vi "Read_INI.vi"(3 "error in (no error)":errorcluster caption="错误输入（无错误）") -> (0 "error out":errorcluster caption="错误输出", 2 "HandsPara":T1)   [LabVIEW 2016]
uses:
  Controls/handspara.ctl
  <vilib>/Utility/config.llb/Read Key (U32).vi
  <vilib>/Utility/config.llb/NI_LVConfig.lvlib
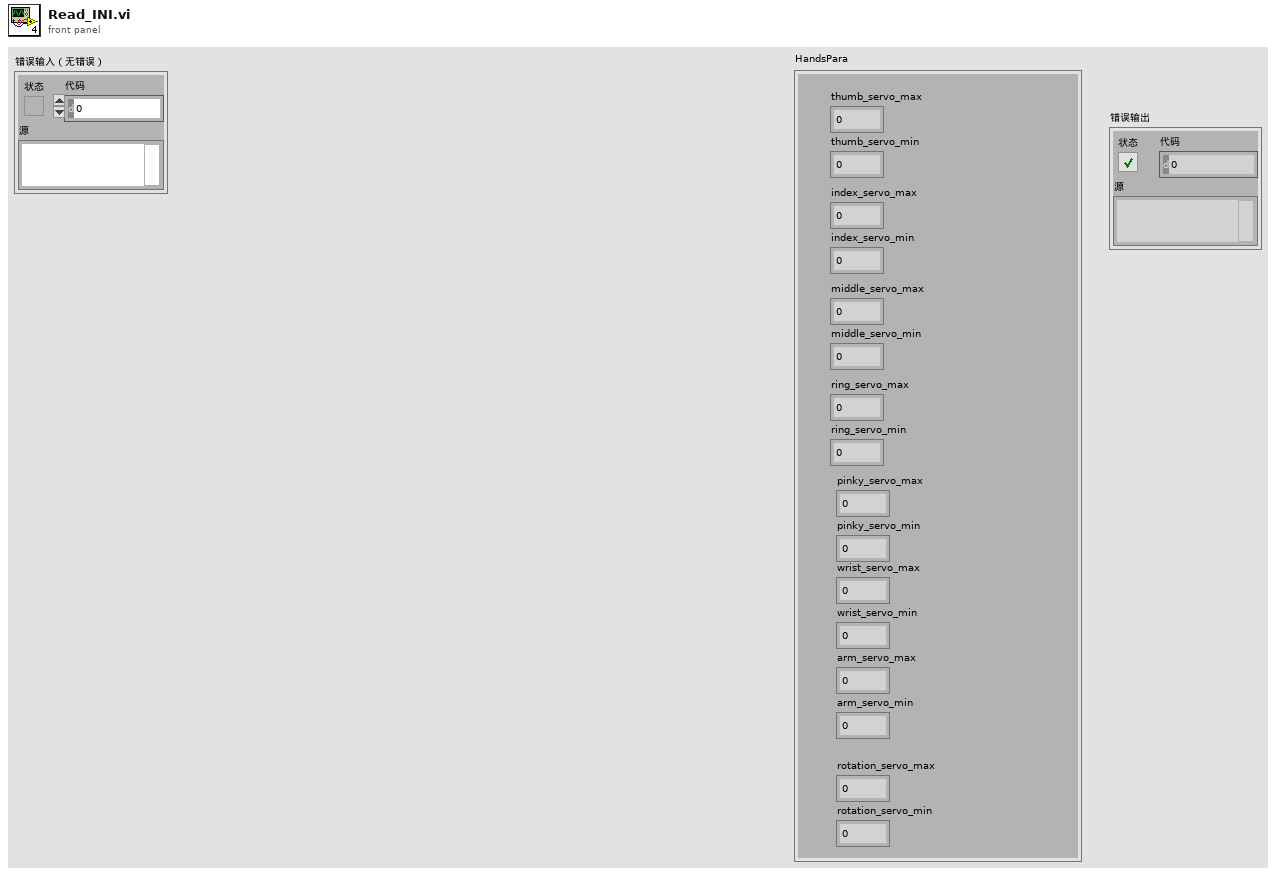
[diagram p1: front panel]
types:
  T1 = typedef "handspara.ctl" = cluster{"thumb_servo_max":u32, "thumb_servo_min":u32, "index_servo_max ":u32, "index_servo_min":u32, "middle_servo_max ":u32, "middle_servo_min":u32, "ring_servo_max":u32, "ring_servo_min":u32, "pinky_servo_max ":u32, "pinky_servo_min ":u32, "wrist_servo_max":u32, "wrist_servo_min":u32, "arm_servo_max ":u32, "arm_servo_min":u32, "rotation_servo_max ":u32, "rotation_servo_min ":u32}
  T2 = typedef "NI_LVConfig.lvlib/Config Data RefNum.ctl" = refnum<k1>
  T3 = cluster{"[0]":u32, "[1]":u32, "[2]":u32, "[3]":u32, "[4]":u32, "[5]":u32, "[6]":u32, "[7]":u32, "[8]":u32, "[9]":u32, "[10]":u32, "[11]":u32, "[12]":u32, "[13]":u32, "[14]":u32, "[15]":u32}
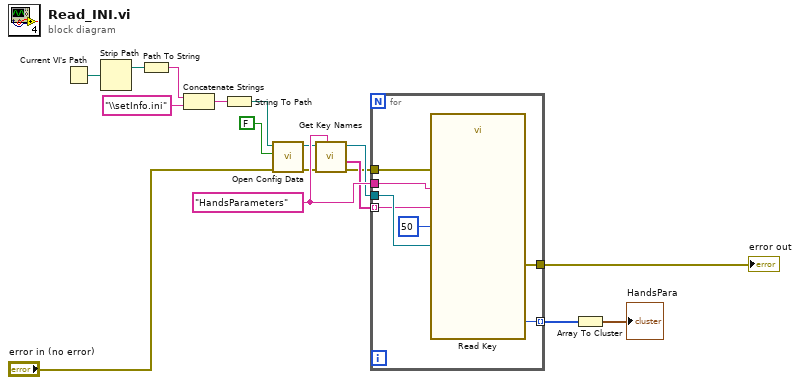
[diagram p0: block diagram]
diagram:
  w10 = "HandsParameters" ("section")
  n1 = Current VI's Path() -> (path=w15:path)
  n2 = Strip Path(path=w15) -> (stripped path=w14:path)  [unwired: 1 out]
  n3 = Path To String(path=w14) -> (string=w17:string)
  n4 = Concatenate Strings(w17, "\\setInfo.ini" ("string")) -> (w16:string)
  n5 = String To Path(string=w16) -> (path=w11:path)
  n6 = call <vilib>:"Open Config Data.vi"("error in (no error)"="error in (no error)", "create file if necessary (T)"=FALSE, "configuration file path"=w11) -> ("error out"=w6:errorcluster, "refnum"=w8:T2)  [unwired: 6 in, 1 out]
  n7 = call <vilib>:"Get Key Names.vi"("section"=w10, "error in (no error)"=w6, "refnum"=w8) -> ("error out"=w5:errorcluster, "key names"=w9:string[], "refnum out"=w7:T2)  [unwired: 5 in, 1 out]
  n8 = for {
    tunnel: w10 -> [w23]
    tunnel: w9 -> [w20] mode=indexing
    tunnel: w7 -> [w22]
    tunnel: w5 -> [w21]
    tunnel: [w19] -> w4 mode=indexing
    tunnel: [w18] -> w2
    n9 = call-poly <vilib>:"Read Key.vi"("section"=w23, "error in (no error)"=w21, "default value"=u32 50, "key"=w20, "refnum"=w22) -> ("error out"=w18:errorcluster, "value"=w19:u32)  [unwired: 3 in, 2 out]
  }
  "error out" <- w2
  n10 = Array To Cluster(array=w4) -> (cluster=→"HandsPara":T3)
